vi "Build Virtual Path.vi"(0 "ProjItem* in":refnum<vi>, 1 "VI ProjPath in":string, 2 "Top Level Name":string="My Computer", 3 "error in (no error)":errorcluster) -> (7 "ProjItem* out":refnum<vi>, 8 "VI ProjPath out":string, 10 "error out":errorcluster)   [LabVIEW 2013, in "SET Project Editor.lvlib"]
doc: "Build Virtual Path.vi\n\nRecursive function builds the virtual path of a project item\nup to the top level."
uses:
  SET Project Editor.lvlib
panel:
  # "Build Virtual Path.vi\n\nRecursive function builds the virtual path of a project item\nup to the top level."
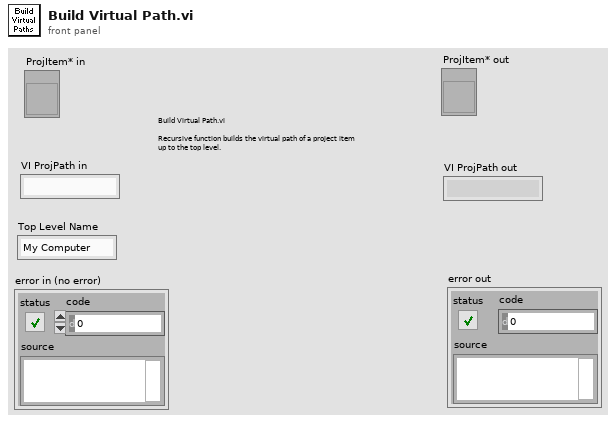
[diagram p1: front panel]
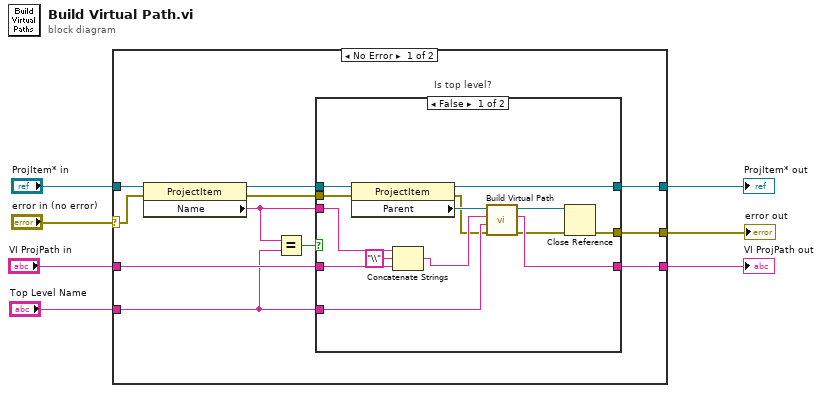
[diagram p0: block diagram]
diagram:
  n1 = case shown="No Error" "error in (no error)" {
    selector: "error in (no error)" -> [w8 w38]
    tunnel: "ProjItem* in" -> [w18 w37]
    tunnel: "VI ProjPath in" -> [w15 w36]
    tunnel: [w14 w37] -> w5
    tunnel: [w13 w36] -> w4
    tunnel: "Top Level Name" -> [w11 _]
    tunnel: [w9 w38] -> w2
    frame No Error {
      # "Is top level?"
      n2 = property class="ProjectItem"(reference=w18, error in=w8) -> (reference out=w16:refnum<vi>, error out=w10:errorcluster, "Name"=w12:string)
      n3 = Equal?(x=w12, y=w11) -> (x = y?=w17:bool)
      n4 = case shown="False" w17 {
        tunnel: w16 -> [w29 w35]
        tunnel: w15 -> [w31 w33]
        tunnel: [w25 w33] -> w13
        tunnel: [w28 w35] -> w14
        tunnel: w12 -> [w30 _]
        tunnel: w11 -> [w24 _]
        tunnel: w10 -> [w23 w34]
        tunnel: [w22 w34] -> w9
        frame False {
          n5 = property class="ProjectItem"(reference=w29, error in=w23) -> (reference out=w28:refnum<vi>, error out=w21:errorcluster, "Parent"=w27:refnum<vi>)
          n6 = Concatenate Strings(w30, "\\" ("string"), w31) -> (w26:string)
          n7 = call "Build Virtual Path.vi"("ProjItem* in"=w27, "VI ProjPath in"=w26, "Top Level Name"=w24, "error in (no error)"=w21) -> ("ProjItem* out"=w19:refnum<vi>, "VI ProjPath out"=w25:string, "error out"=w20:errorcluster)  [unwired: 4 in]
          n8 = Close Reference(reference=w19, error in (no error)=w20) -> (error out=w22:errorcluster)
        }
        frame True {
        }
      }
    }
    frame Error {
    }
  }
  "ProjItem* out" <- w5
  "VI ProjPath out" <- w4
  "error out" <- w2
